vi "factorial_for_n.vi"() -> ()   [LabVIEW 2019]
panel:
  in  "?":bool
  out "S.O.F":dbl
  in  "INPUT":dbl
  # "Sum of Factorial"
  # "="
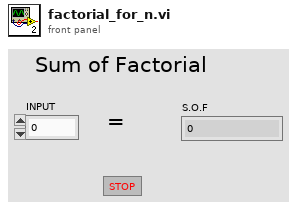
[diagram p1: front panel]
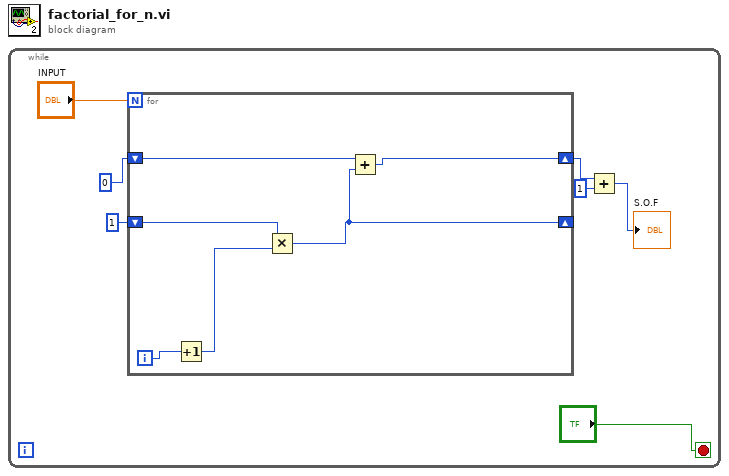
[diagram p0: block diagram]
diagram:
  n1 = while {
    stop <- "?" stop-if-true
    n2 = for {
      N: "INPUT" -> [_]
      shift-right: [w8] -> _
      shift-left: 1 -> [w11]
      shift-right: [w10] -> w4
      shift-left: 0 -> [w9]
      i -> [w13]
      n3 = Increment(x=w13) -> (x+1=w12:i32)
      n4 = Multiply(x=w11, y=w12) -> (x*y=w8:i32)
      n5 = Add(x=w9, y=w8) -> (x+y=w10:i32)
    }
    n6 = Add(x=w4, y=1) -> (x+y=→"S.O.F":i32)
  }
